vi "Receive.vi"(8 "error in (no error)":errorcluster, 11 "Framework in":refnum<class "Framework.lvclass">) -> (0 "error out":errorcluster, 3 "Framework out":refnum<class "Framework.lvclass">)   [LabVIEW 2017, in "DSF Core.lvlib" / "Framework.lvclass"]
uses:
  Framework.lvclass
  Framework.lvclass/Framework.ctl
  Performance/Performance.lvclass/Performance.ctl
  Plugin/Plugin.lvclass/Plugin.ctl
  Transfer Group/Transfer Group.lvclass/Transfer Group.ctl
  Timing/Timing.lvclass/Timing.ctl
  Interfaces/Interface/Interface.lvclass/Interface.ctl
  Buffers/Buffers.lvclass/Buffers.ctl
  <vilib>/NI/Memory Manager/Classes/Pointer/Pointer.lvclass/Pointer.ctl
  Transfer Group/Wait For Previous.vi
  Transfer Group/Update Status.vi
  Transfer Group/Increment Iteration.vi
  Transfer Group/Get Iteration.vi
  Dispatcher/Dispatch Transfer Group.vi
  Transfer Group/Get ID.vi
  Transfer Group/Copy Async to Inline.vi
  Transfer Group/Get Active.vi
  Plugin/Get ID.vi
  Transfer Group/Retrieve from FIFO.vi
  Transfer Group Status/Write Status.vi
  Timing/Increment Iteration.vi
  Timing/Get Iteration.vi
  Interfaces/Dispatcher/Send Dispatcher Command.vi
  Buffers/Copy Async to Inline.vi
  Transfer Group/Read Return FIFO.vi
  Transfer Group/Increment Late Count.vi
  <vilib>/NI/Memory Manager/Classes/Pointer/Get Address.vi
  Transfer Group Status/Status Size.vi
  <vilib>/NI/Memory Manager/Classes/Pointer/Check Null Pointer.vi
  <vilib>/NI/Memory Manager/Classes/Pointer/Check Size (0D).vi
  Interfaces/Dispatcher/Write.vi
  Interfaces/Dispatcher/Write Dispatcher Command.vi
  <vilib>/NI/Memory Manager/Classes/Pointer/Copy All.vi
  <vilib>/NI/Memory Manager/Classes/Pointer/Errors.vi
  <vilib>/NI/Memory Manager/Classes/Pointer/Null Pointer.vi
  <vilib>/NI/Memory Manager/Classes/Pointer/Is Null.vi
  <vilib>/NI/Memory Manager/Classes/Pointer/Out of Bounds.vi
  <vilib>/NI/Memory Manager/Classes/Pointer/Get Size.vi
  Interfaces/Interface/Send Command.vi
  <vilib>/NI/Memory Manager/Classes/Pointer/Copy.vi
  <vilib>/NI/Memory Manager/Classes/Pointer/Create Error.vi
  <vilib>/NI/Memory Manager/VIs/Source.Write.String.vi
  <vilib>/NI/Memory Manager/Classes/Pointer/Write Pointer Size.vi
  <vilib>/NI/Memory Manager/VIs/Source.Write.Scalar.Base10.vi
  <vilib>/NI/Memory Manager/VIs/Source.Write.Scalar.Base10 (U64).vi
  Interfaces/Interface/Write RT FIFO.vi
  <vilib>/NI/Memory Manager/Classes/Pointer/Copy (No Check).vi
  <vilib>/NI/Memory Manager/Classes/Pointer/Check Pointer Bounds.vi
  <vilib>/NI/Memory Manager/VIs/New Error Cluster Constant.vi
  <vilib>/NI/Memory Manager/VIs/New Error Cluster Constant (512B).vi
  <vilib>/NI/Memory Manager/VIs/Error Cluster.Set Status.vi
  <vilib>/NI/Memory Manager/VIs/Error Cluster.Set Code.vi
  <vilib>/NI/Memory Manager/VIs/Error Cluster.Set VI Source.vi
  <vilib>/NI/Memory Manager/Constants/Constants.vi
  <vilib>/NI/Memory Manager/Constants/Library Name.vi
  <vilib>/NI/Memory Manager/Classes/Pointer/Pointer Error Info.vi
  <vilib>/NI/Memory Manager/Constants/Pointer Class Name.vi
  Interfaces/Dispatcher/Dispatcher Interface.lvclass
  C:/Git/DSF/Data Sharing Framework/Source/Core/Classes/Interfaces/Interface/Interface.lvclass
  Buffer/Buffer.lvclass
  C:/Program Files (x86)/National Instruments/LabVIEW 2017/vi.lib/NI/Memory Manager/Classes/Pointer/Pointer.lvclass
  Transfer Group Status/Status.lvclass
  Transfer Group/Errors.vi
  Transfer Group/Return Timeout Error.vi
  Transfer Group/Invalid Iteration Error.vi
  Interfaces/Interface/Errors.vi
  Interfaces/Dispatcher/Command Timeout.vi
  VIs/VI Name.vi
  Interfaces/Dispatcher/Class Name.vi
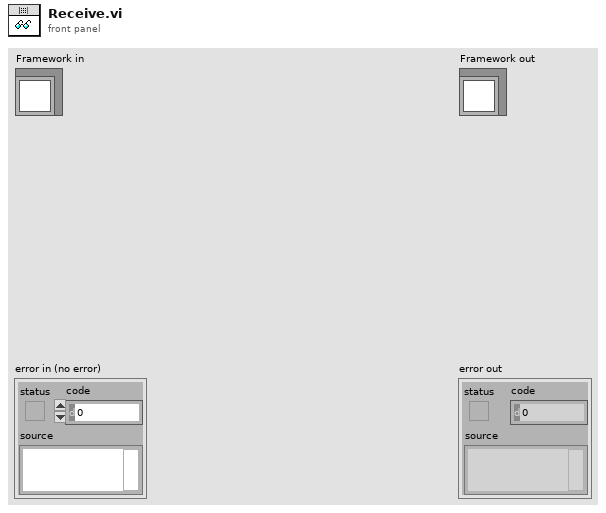
[diagram p1: front panel]
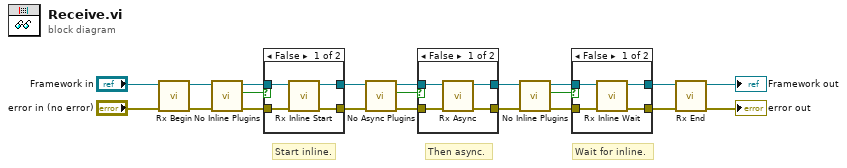
[diagram p0: block diagram]
diagram:
  # "Wait for inline."
  # "Start inline."
  # "Then async."
  n1 = call "Rx Begin.vi"("error in (no error)"="error in (no error)", "Framework in"="Framework in") -> ("error out"=w4:errorcluster, "Framework out"=w3:refnum<class "Framework.lvclass">)  [unwired: 8 in]
  n2 = call "No Inline Plugins.vi"("error in (no error)"=w4, "Framework in"=w3) -> ("error out"=w16:errorcluster, "no inline?"=w13:bool, "Framework out"=w17:refnum<class "Framework.lvclass">)  [unwired: 7 in]
  n3 = case shown="False" w13 {
    tunnel: w17 -> [w25 w27]
    tunnel: w16 -> [w24 w26]
    tunnel: [w23 w27] -> w15
    tunnel: [w22 w26] -> w14
    frame False {
      n4 = call "Rx Inline Start.vi"("error in (no error)"=w24, "Framework in"=w25) -> ("error out"=w22:errorcluster, "Framework out"=w23:refnum<class "Framework.lvclass">)  [unwired: 8 in]
    }
    frame True {
    }
  }
  n5 = call "No Async Plugins.vi"("error in (no error)"=w14, "Framework in"=w15) -> ("error out"=w12:errorcluster, "no async?"=w10:bool, "Framework out"=w11:refnum<class "Framework.lvclass">)  [unwired: 7 in]
  n6 = case shown="False" w10 {
    tunnel: w11 -> [w31 w33]
    tunnel: w12 -> [w30 w32]
    tunnel: [w29 w33] -> w6
    tunnel: [w28 w32] -> w5
    frame False {
      n7 = call "Rx Async.vi"("error in (no error)"=w30, "Framework in"=w31) -> ("error out"=w28:errorcluster, "Framework out"=w29:refnum<class "Framework.lvclass">)  [unwired: 8 in]
    }
    frame True {
    }
  }
  n8 = call "No Inline Plugins.vi"("error in (no error)"=w5, "Framework in"=w6) -> ("error out"=w9:errorcluster, "no inline?"=w7:bool, "Framework out"=w8:refnum<class "Framework.lvclass">)  [unwired: 7 in]
  n9 = case shown="False" w7 {
    tunnel: w8 -> [w37 w39]
    tunnel: w9 -> [w36 w38]
    tunnel: [w35 w39] -> w1
    tunnel: [w34 w38] -> w2
    frame False {
      n10 = call "Rx Inline Wait.vi"("error in (no error)"=w36, "Framework in"=w37) -> ("error out"=w34:errorcluster, "Framework out"=w35:refnum<class "Framework.lvclass">)  [unwired: 8 in]
    }
    frame True {
    }
  }
  n11 = call "Rx End.vi"("error in (no error)"=w2, "Framework in"=w1) -> ("error out"=→"error out":errorcluster, "Framework out"=→"Framework out":refnum<class "Framework.lvclass">)  [unwired: 8 in]
